vi "Example.vi"() -> ()   [LabVIEW 2019, in "Sprite.lvlib"]
uses:
  Sprite.lvlib
  SpriteData.ctl
  <vilib>/Platform/TimedLoop/XDataNode/timing_clust.ctl
  <vilib>/Platform/TimedLoop/XDataNode/nitl_modes.ctl
  <vilib>/Platform/TimedLoop/XDataNode/wakeup.ctl
  <vilib>/rvi/Emulation/niFpgaGetClockAttributes.vi
  <vilib>/rvi/Emulation/niFpgaSctlEmulationGetInTimedLoop.vi
  <vilib>/rvi/Emulation/niFpgaEmulationReportErrorSimple.vi
  <vilib>/rvi/Emulation/niFpgaCriticalErrorInLSC.vi
  <vilib>/rvi/Memory/Memory_Emulation/nirvimemoryFastEmulation.vi
  <vilib>/rvi/Memory/Memory_Emulation/nirvimemoryEmulation.vi
  <vilib>/rvi/Emulation/niFpgaEmulationIsFPGAContextNoSignature.vi
  <vilib>/rvi/DataTransferAndStorage/Container/Common/niFpgaContainerGetUniqueNameForEmu.vi
  <vilib>/rvi/Emulation/niFpgaProcessEmulError.vi
  <vilib>/rvi/errors/nirviReportUnexpectedCaseInternalError (U32).vi
  <vilib>/platform/TimedLoop/XDataNode/XDataNode.xnode
  <vilib>/rvi/DataTransferAndStorage/Container/XNode/niFpgaContainer.xnode
  <vilib>/Platform/TimedLoop/XDataNode/XDNodeRunTimeDep.lvlib
  Shared/Shared.lvlib
  VGA/VGA.lvlib
panel:
  in  "SpritesData":T1[](array[typedef])=[{"Pos_X"=0, "Pos_Y"=0, "Width"=0, "Height"=0, "BufferIndex"=0, "TransparencyColor"=0.0}, {"Pos_X"=0, "Pos_Y"=0, "Width"=0, "Height"=0, "BufferIndex"=0, "TransparencyColor"=0.0}, {"Pos_X"=0, "Pos_Y"=0, "Width"=0, "Height"=0, "BufferIndex"=0, "TransparencyColor"=0.0}]
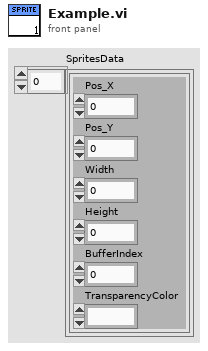
[diagram p1: front panel]
types:
  T1 = typedef "Sprite.lvlib/SpriteData.ctl" = cluster{"Pos_X":u16, "Pos_Y":u16, "Width":u8, "Height":u8, "BufferIndex":u16, "TransparencyColor":fxp<+,3,3>}
  T2 = typedef "XDNodeRunTimeDep.lvlib/timing_clust.ctl" = cluster{"Expected End [f-1]":u64, "Actual End [f-1]":u64, "Finished Late? [f-1]":bool, "Expected End [i-1]":u64, "Actual End [i-1]":u64, "Finished Late? [i-1]":bool, "Expected Start [i]":u64, "Actual Start [i]":u64, "Expected Start [f]":u64, "Actual Start [f]":u64, "Source Name":string, "Structure Name":string, "Period":i64, "Deadline":i64, "Offset":i64, "Start":i64, "Priority":i32, "Timeout":i32, "Mode":T3, "Wakeup Reason":T4, "Error":errorcluster, "Source Type":string, "Secondary Source Type":string, "Global End Time":u64, "Global Start Time":u64, "Frame Duration":u64, "Iteration Duration":u64, "Assigned CPU":i32, "I/O Scan Engine Mode":u32}
  T3 = typedef "XDNodeRunTimeDep.lvlib/nitl_modes.ctl" = enum32{"No Change", "Process missed periods, maintain original phase", "Discard missed periods, maintain original phase", "Process missed periods, ignore original phase", "Discard missed periods, ignore original phase"}
  T4 = typedef "XDNodeRunTimeDep.lvlib/wakeup.ctl" = enum32{"Normal", "Aborted", "Asynchronous wakeup", "Timing source error", "Timed loop error", "Timeout"}
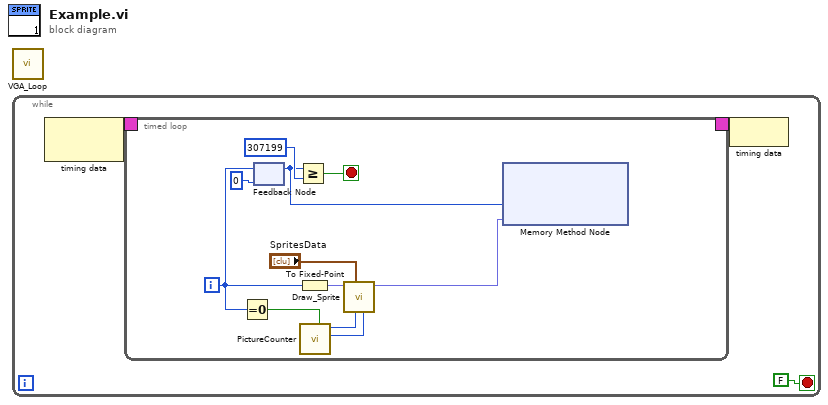
[diagram p0: block diagram]
diagram:
  n1 = call "VGA_Loop.vi"() -> ()  [unwired: 12 in]
  n2 = while {
    stop <- FALSE stop-if-true
    n3 = node-c288() -> (w3:T2)  [unwired: 1 in]
    n4 = timed-loop {
      timing: w3 -> [_]
      timing-out: [_] -> w2
      i -> [w6]
      stop <- w13 stop-if-true
      n5 = Equal To 0?(x=w6) -> (x = 0?=w12:bool)
      n6 = feedback-in #1(w6) -> ()
      n7 = feedback #1(0) -> (w5:i32)
      n8 = Greater Or Equal?(x=w5, y=307199) -> (x >= y?=w13:bool)
      n9 = To Fixed-Point(number=w6) -> (fixed-point=w7:fxp<+,3,3>)  [unwired: 1 in]
      n10 = call "PictureCounter.vi"("Reset? (f)"=w12) -> ("y"=w9:u16, "x"=w10:u16)  [unwired: 9 in]
      n11 = call "Draw_Sprite.vi"("y_index"=w9, "x_index"=w10, "SpritesData"="SpritesData", "color_in"=w7) -> ("color_out"=w11:fxp<+,3,3>)  [unwired: 7 in]
      n12 = xnode ("Memory Method Node")("Address"=w5, "Data"=w11) -> ()  [unwired: 1 in, 1 out]
    }
    n13 = node-c288(w2) -> ()
  }
